vi "Msg LstBox Append.vi"(7 "Show Date in LstBox":bool, 8 "error in (no error)":errorcluster, 9 "File Ref":refnum<file>, 10 "Msg":string, 11 "LstBox Refnum":refnum<vi>) -> (0 "error out":errorcluster)   [LabVIEW 2016, in "Common.lvlib"]
uses:
  <userlib>/Common Components/Common/Common.lvlib
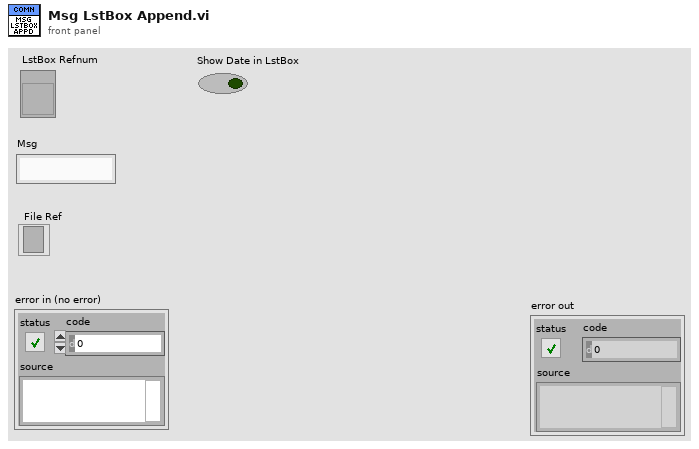
[diagram p1: front panel]
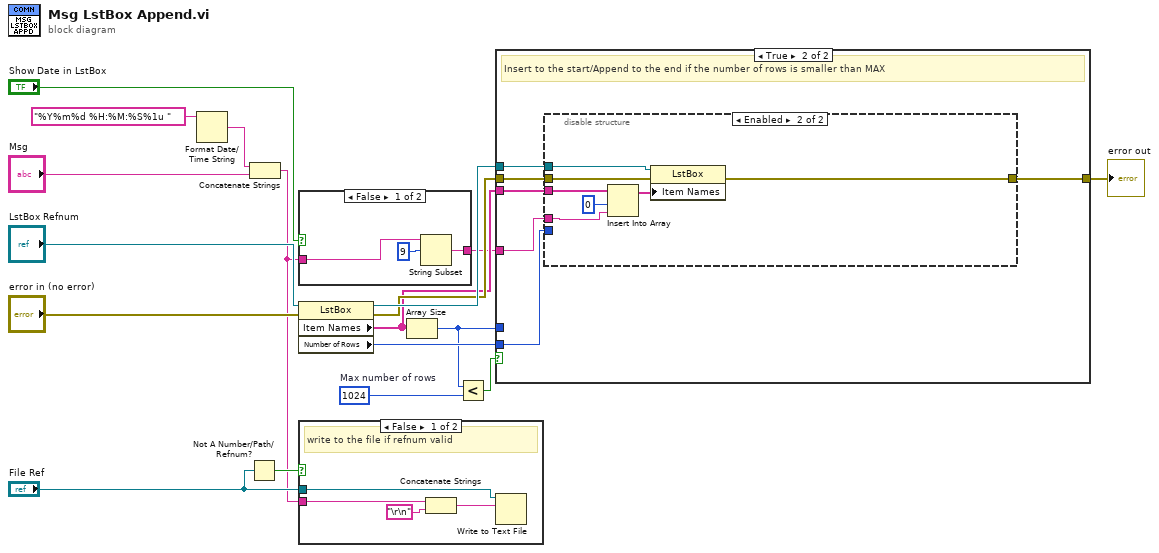
[diagram p0: block diagram]
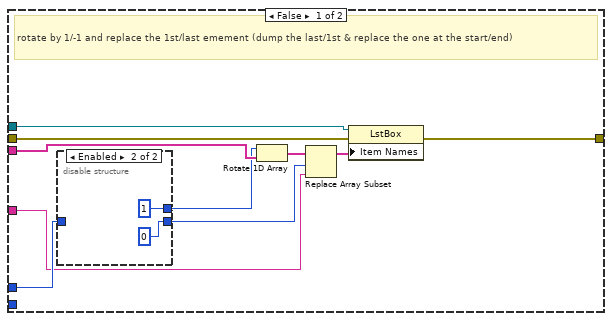
[diagram p4: hidden frame]
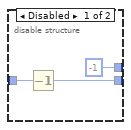
[diagram p5: hidden frame]
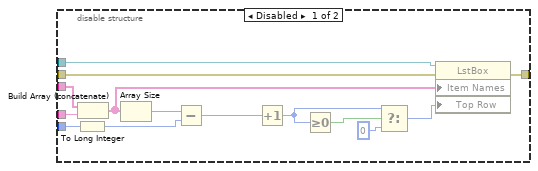
[diagram p6: hidden frame]
diagram:
  w8 = 1024  # Max number of rows
  n1 = Format Date/Time String(time format string (%c)="%Y%m%d %H:%M:%S%1u ") -> (date/time string=w17:string)  [unwired: 2 in]
  n2 = Not A Number/Path/Refnum?(number/path/refnum="File Ref") -> (NaN/Path/Refnum?=w5:bool)
  n3 = Concatenate Strings(w17, "Msg") -> (w2:string)
  n4 = case shown="False" "Show Date in LstBox" {
    tunnel: w2 -> [w21 w22]
    tunnel: [w19 w22] -> w1
    frame False {
      n5 = String Subset(string=w21, offset (0)=9) -> (substring=w19:string)  [unwired: 1 in]
    }
    frame True {
    }
  }
  n6 = property class="LstBox"(reference="LstBox Refnum", error in="error in (no error)") -> (reference out=w15:refnum<vi>, error out=w12:errorcluster, "Item Names"=w9:string[], "Number of Rows"=w10:u32)
  n7 = case shown="False" w5 {
    tunnel: "File Ref" -> [w26 _]
    tunnel: w2 -> [w25 _]
    frame False {
      # "write to the file if refnum valid"
      n8 = Concatenate Strings(w25, "\r\n") -> (w24:string)
      n9 = Write to Text File(file (use dialog)=w26, text=w24) -> ()  [unwired: 2 in, 3 out]
    }
    frame True {
    }
  }
  n10 = Array Size(array=w9) -> (size(s)=w6:i32)
  n11 = Less?(x=w6, y=w8) -> (x < y?=w7:bool)
  n12 = case shown="True" w7 {
    tunnel: w15 -> [w29 w47]
    tunnel: w1 -> [w31 w46]
    tunnel: w12 -> [w28 w45]
    tunnel: [w27 w44] -> w11
    tunnel: w10 -> [_ w43]
    tunnel: w9 -> [w36 w42]
    tunnel: w6 -> [w33 _]
    frame False {
      # "rotate by 1/-1 and replace the 1st/last emement (dump the last/1st & replace the one at the start/end)"
      n13 = disable-structure shown="Enabled" {
        disable-tunnel: [-1 1] -> w35
        disable-tunnel: w33 -> [w38 _]
        disable-tunnel: [w37 0] -> w32
        frame Disabled {
          n14 = Decrement(x=w38) -> (x-1=w37:i32)
        }
        frame Enabled {
        }
      }
      n15 = Rotate 1D Array(1:w36, 2:w35) -> (0:w34:string[])
      n16 = Replace Array Subset(array=w34, new element=w31, index=w32) -> (w30:string[])
      n17 = property class="LstBox"(reference=w29, error in=w28, "Item Names"=w30) -> (error out=w27:errorcluster)  [unwired: 1 out]
    }
    frame True {
      # "Insert to the start/Append to the end if the number of rows is smaller than MAX"
      n18 = disable-structure shown="Enabled" {
        disable-tunnel: w47 -> [w61 w68]
        disable-tunnel: w46 -> [w60 w63]
        disable-tunnel: w45 -> [w59 w66]
        disable-tunnel: [w58 w67] -> w44
        disable-tunnel: w43 -> [w55 _]
        disable-tunnel: w42 -> [w48 w65]
        frame Disabled {
          n19 = To Long Integer(number=w55) -> (32bit integer=w50:i32)
          n20 = Build Array (concatenate)(w48, w60) -> (w56:string[])
          n21 = Array Size(array=w56) -> (size(s)=w57:i32)
          n22 = Subtract(x=w57, y=w50) -> (x-y=w53:i32)
          n23 = Increment(x=w53) -> (x+1=w49:i32)
          n24 = Greater Or Equal To 0?(x=w49) -> (x >= 0?=w52:bool)
          n25 = Select(t=w49, s=w52, f=u32 0) -> (s? t:f=w54:u32)
          n26 = property class="LstBox"(reference=w61, error in=w59, "Item Names"=w56, "Top Row"=w54) -> (error out=w58:errorcluster)  [unwired: 1 out]
        }
        frame Enabled {
          n27 = Insert Into Array(array=w65, index=0, new element=w63) -> (w62:string[])
          n28 = property class="LstBox"(reference=w68, error in=w66, "Item Names"=w62) -> (error out=w67:errorcluster)  [unwired: 1 out]
        }
      }
    }
  }
  "error out" <- w11
